vi "加标回收停止对话框.vi"() -> (2 "数组":bool[](array[boolean]), 3 "check？":bool)   [LabVIEW 2016, in "质控单元V2.lvlib"]
panel:
  in  "采配水":bool caption="启用"
  in  "取消":bool
  in  "确认":bool
  in  "CODCr":bool caption="启用"
  in  "CODMn":bool caption="启用"
  in  "总氮":bool caption="启用"
  in  "总磷":bool caption="启用"
  in  "氨氮":bool caption="启用"
  # "请选择要停止的参数"
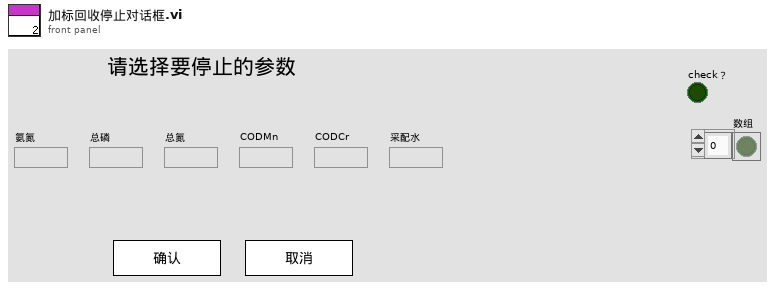
[diagram p1: front panel]
types:
  T1 = cluster{"氨氮":bool, "总磷":bool, "总氮":bool, "CODMn":bool, "CODCr":bool}
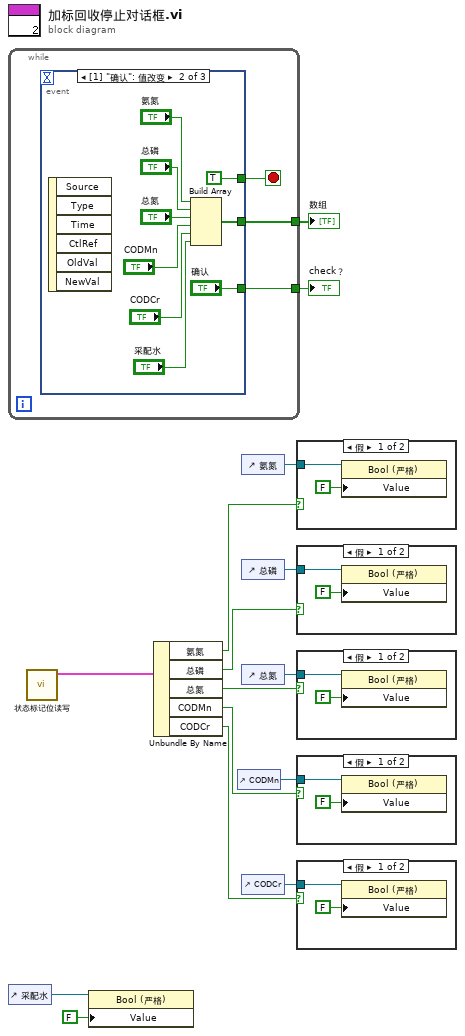
[diagram p0: block diagram]
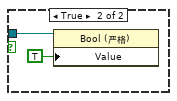
[diagram p2: hidden frame]
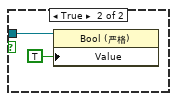
[diagram p3: hidden frame]
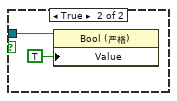
[diagram p4: hidden frame]
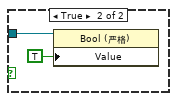
[diagram p5: hidden frame]
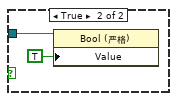
[diagram p6: hidden frame]
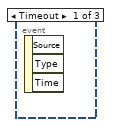
[diagram p7: hidden frame]
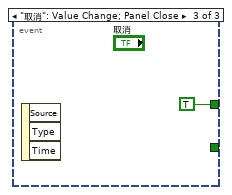
[diagram p8: hidden frame]
diagram:
  n1 = while {
    tunnel: [w17] -> w3
    tunnel: [w16] -> w2
    stop <- w18 stop-if-true
    n2 = event shown="[1] \"确认\": 值改变" {
      selector: _ -> [_ _ _]
      dyn-events: _ -> [_ _ _]
      timeout: _ -> [_ _ _]
      tunnel: [_ TRUE TRUE] -> w18
      tunnel: [_ w21 _] -> w17
      tunnel: [_ "确认" _] -> w16
      event Timeout {
        n3 = event-data() -> ()  [unwired: 1 in, 3 out]
      }
      event "确认": Value Change {
        n4 = event-data() -> ()  [unwired: 1 in, 6 out]
        n5 = Build Array("氨氮", "总磷", "总氮", "CODMn", "CODCr", "采配水") -> (w21:bool[])
      }
      event "取消": Value Change; Panel Close {
        n6 = event-data() -> ()  [unwired: 1 in, 3 out]
      }
    }
  }
  "数组" <- w3
  "check？" <- w2
  n7 = control-ref of="采配水"() -> (w4:refnum<vi>)
  n8 = call "状态标记位读写.vi"() -> ("运维标记位"=w1:T1)  [unwired: 11 in]
  n9 = property class="Bool (严格)"(reference=w4, "Value"=FALSE ("值")) -> ()  [unwired: 1 in, 2 out]
  n10 = Unbundle By Name(w1) -> ("氨氮"=w15:bool, "总磷"=w14:bool, "总氮"=w13:bool, "CODMn"=w12:bool, "CODCr"=w11:bool)
  n11 = control-ref of="CODMn"() -> (w7:refnum<vi>)
  n12 = control-ref of="氨氮"() -> (w10:refnum<vi>)
  n13 = control-ref of="总磷"() -> (w9:refnum<vi>)
  n14 = control-ref of="总氮"() -> (w8:refnum<vi>)
  n15 = control-ref of="CODCr"() -> (w6:refnum<vi>)
  n16 = case shown="假" w15 {
    tunnel: w10 -> [w30 w32]
    frame False {
      n17 = property class="Bool (严格)"(reference=w30, "Value"=FALSE ("值")) -> ()  [unwired: 1 in, 2 out]
    }
    frame True {
      n18 = property class="Bool (严格)"(reference=w32, "Value"=TRUE ("值")) -> ()  [unwired: 1 in, 2 out]
    }
  }
  n19 = case shown="假" w14 {
    tunnel: w9 -> [w34 w36]
    frame False {
      n20 = property class="Bool (严格)"(reference=w34, "Value"=FALSE ("值")) -> ()  [unwired: 1 in, 2 out]
    }
    frame True {
      n21 = property class="Bool (严格)"(reference=w36, "Value"=TRUE ("值")) -> ()  [unwired: 1 in, 2 out]
    }
  }
  n22 = case shown="假" w13 {
    tunnel: w8 -> [w38 w40]
    frame False {
      n23 = property class="Bool (严格)"(reference=w38, "Value"=FALSE ("值")) -> ()  [unwired: 1 in, 2 out]
    }
    frame True {
      n24 = property class="Bool (严格)"(reference=w40, "Value"=TRUE ("值")) -> ()  [unwired: 1 in, 2 out]
    }
  }
  n25 = case shown="假" w12 {
    tunnel: w7 -> [w42 w44]
    frame False {
      n26 = property class="Bool (严格)"(reference=w42, "Value"=FALSE ("值")) -> ()  [unwired: 1 in, 2 out]
    }
    frame True {
      n27 = property class="Bool (严格)"(reference=w44, "Value"=TRUE ("值")) -> ()  [unwired: 1 in, 2 out]
    }
  }
  n28 = case shown="假" w11 {
    tunnel: w6 -> [w46 w48]
    frame False {
      n29 = property class="Bool (严格)"(reference=w46, "Value"=FALSE ("值")) -> ()  [unwired: 1 in, 2 out]
    }
    frame True {
      n30 = property class="Bool (严格)"(reference=w48, "Value"=TRUE ("值")) -> ()  [unwired: 1 in, 2 out]
    }
  }
